vi "Discover_MXA.vi"(8 "error in":errorcluster {"code" format="%.0x"}, 11 "Session In":refnum<visa-resource-name>="TCPIP0::10.0.1.24::inst0::INSTR") -> (0 "error out":errorcluster {"code" format="%.0x"}, 2 "Success?(t)":bool, 3 "Session Out":refnum<visa-resource-name>, 5 "Model_Out":string, 7 "IsPSA?(t)":bool)   [LabVIEW 2018]
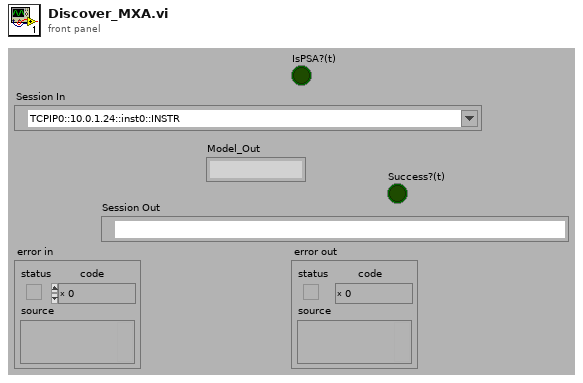
[diagram p1: front panel]
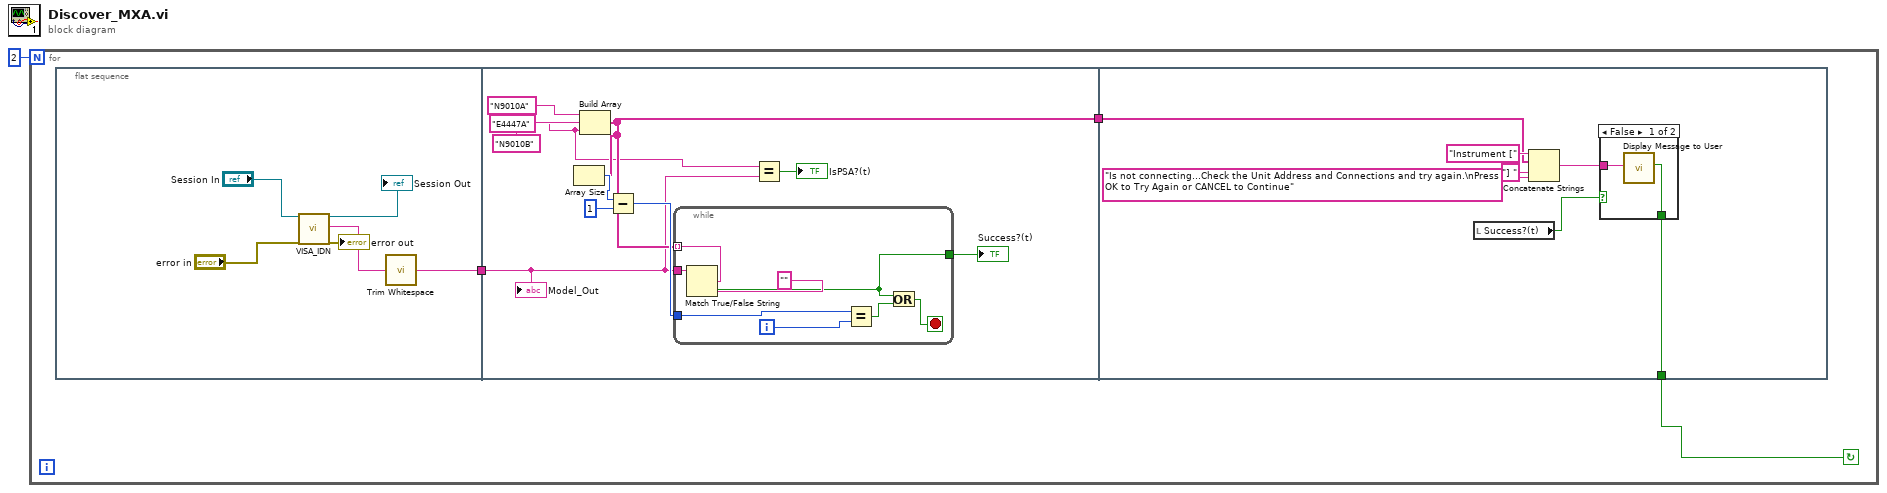
[diagram p0: block diagram]
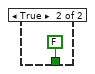
[diagram p2: hidden frame]
diagram:
  n1 = for {
    N: 2 -> [_]
    stop <- w2 continue-if-true
    n2 = flat-sequence {
      tunnel: [w7] -> w4
      tunnel: w4 -> [w12]
      tunnel: [w16] -> w3
      tunnel: w3 -> [w34]
      tunnel: [w29] -> w2
      frame #0 {
        n3 = call "VISA_IDN.vi"("Session In"="Session In", "error in"="error in") -> ("Session Out"=→"Session Out":refnum<visa-resource-name>, "Model"=w10:string, "error out"=→"error out":errorcluster)  [unwired: 11 in, 4 out]
        n4 = call <vilib>:"Trim Whitespace.vi"("string"=w10) -> ("trimmed string"=w7:string)  [unwired: 1 in]
      }
      frame #1 {
        w13 = "E4447A" ("element")
        n5 = Build Array("N9010A" ("element"), "N9010B" ("true string"), w13) -> (w16:string[])
        n6 = Array Size(array=w16) -> (size(s)=w19:i32)
        n7 = Subtract(x=w19, y=1) -> (x-y=w17:i32)
        n8 = while {
          tunnel: w16 -> [w27] mode=indexing
          tunnel: w12 -> [w26]
          tunnel: [w25] -> w20
          tunnel: w17 -> [w21]
          i -> [w22]
          stop <- w24 stop-if-true
          n9 = Match True/False String(2:"" ("false string"), 3:w27, 4:w26) -> (0:w25:bool)  [unwired: 1 out]
          n10 = Equal?(x=w21, y=w22) -> (x = y?=w23:bool)
          n11 = Or(x=w25, y=w23) -> (x .or. y?=w24:bool)
        }
        "Success?(t)" <- w20
        n12 = Equal?(x=w13, y=w12) -> (x = y?=→"IsPSA?(t)":bool)
        "Model_Out" <- w12
      }
      frame #2 {
        n13 = local read "Success?(t)"() -> (w30:bool)
        n14 = Concatenate Strings("Instrument [" ("string"), w34, "] " ("string"), "Is not connecting...Check the Unit Address and Connections and try again.\nPress OK to Try Again or CANCEL to Continue" ("string")) -> (w31:string)
        n15 = case shown="False" w30 {
          tunnel: w31 -> [w37 _]
          tunnel: [w36 FALSE ("OK")] -> w29
          frame False {
            n16 = call "Display Message to User"("Message"=w37) -> ("OK"=w36:bool)  [unwired: 9 in, 1 out]
          }
          frame True {
          }
        }
      }
    }
  }
